vi "LeCroy Wave Series Acquire Waveform With Preview.vi"() -> ()   [LabVIEW 2018]
doc: "This example shows how to use advanced waveform readout parameters. The Preview Waveform Data graph shows signal decimated based on First Point, Sparsing and Number Of Points parameters. The Full Waveform Data graph shows full data as they were acquired by the instrument.\nObserve the time it takes to download the preview data and the full data."
uses:
  LeCroy Wave Series.lvlib
panel:
  in  "Number Of Points (0: all points)":i32
  in  "First Point (0: first point)":i32
  out "Full Download Time":u32
  out "Full Waveform Data":waveform(dbl)(graph)
  in  "Sparsing (1000)":i32=1000
  out "Preview Download Time":u32
  in  "Maximum Sample Points (1M)":i32(ring)=1000000 items=["50"=50, "100"=100, "250"=250, "500"=500, "1000"=1000, "2500"=2500, "5K"=5000, "10K"=10000, "25K"=25000, "50K"=50000, "100K"=100000, "250K"=250000, "500K"=500000, "1M"=1000000]
  in  "Vertical Coupling (0: A1M)":u16(ring) items=["A1M", "D1M", "D50", "Ground"]
  in  "Probe Attenuation (-1)":dbl=-1.0
  in  "Vertical Range (1.0 V)":dbl=10.0
  in  "Timebase (0.0005 s)":dbl=0.0005
  out "Preview Waveform Data":waveform(dbl)(graph)
  in  "Source (0: Channel 1)":u16(ring) items=["Channel 1", "Channel 2", "Channel 3", "Channel 4"]
  in  "VISA resource name":refnum<visa-resource-name>
  # "(c) 2005 - 2012 NATIONAL INSTRUMENTS.  ALL RIGHTS RESERVED."
  # "Note:\nThis VI will time out without acquiring any data if the input signal on channel 1 does not cross 0 V trigger level with positive slope.\nFor more details on triggering pleas see the Edge Triggered Acquisition Example VI."
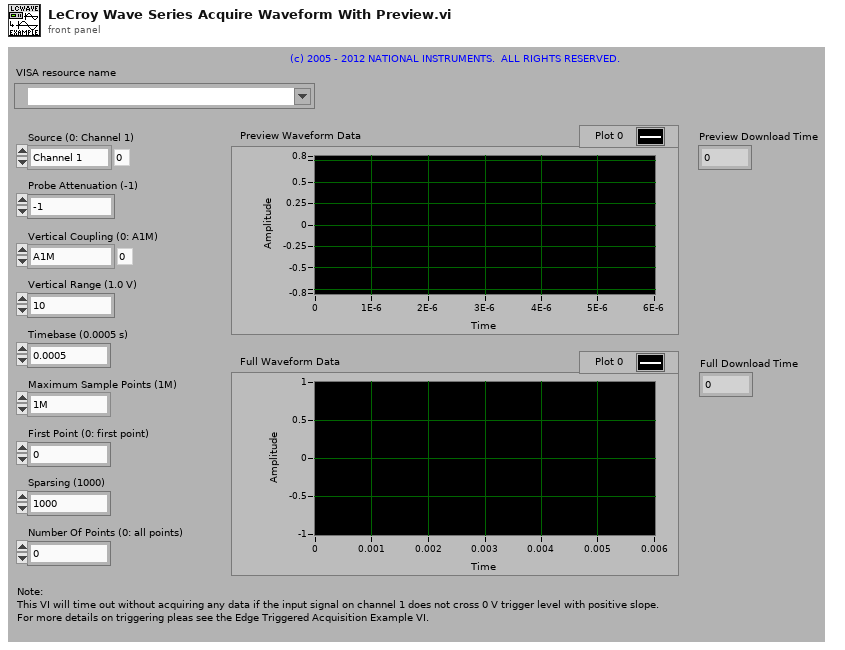
[diagram p1: front panel]
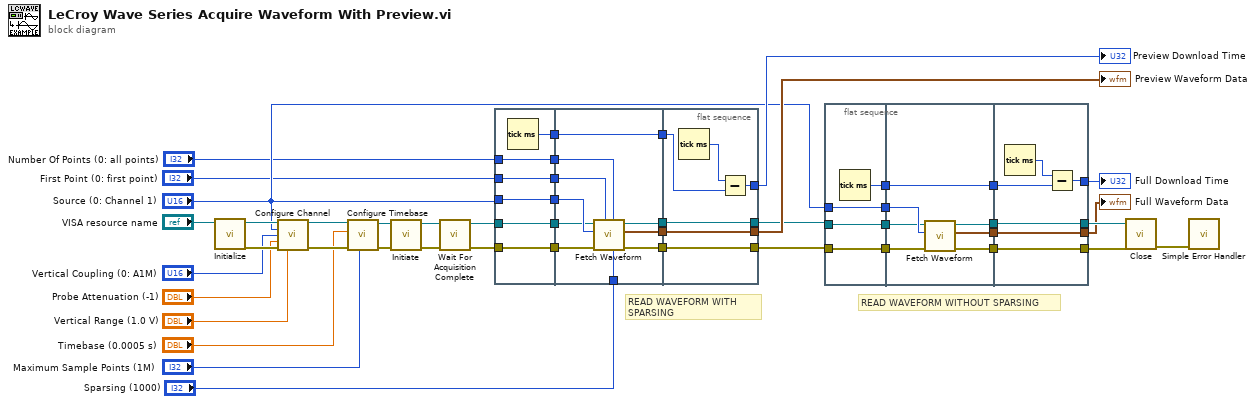
[diagram p0: block diagram]
diagram:
  # "READ WAVEFORM WITHOUT SPARSING"
  # "READ WAVEFORM WITH SPARSING"
  n1 = call "Initialize.vi"("VISA resource name"="VISA resource name") -> ("error out"=w41:errorcluster, "VISA resource name out"=w42:refnum<visa-resource-name>)  [unwired: 9 in]
  n2 = call "Configure Channel.vi"("VISA resource name"=w42, "Channel (0: Channel 1)"="Source (0: Channel 1)", "Vertical Coupling (0: A1M)"="Vertical Coupling (0: A1M)", "Probe Attenuation (-1.0)"="Probe Attenuation (-1)", "error in (no error)"=w41, "Vertical Range (10.0 V)"="Vertical Range (1.0 V)") -> ("VISA resource name out"=w45:refnum<visa-resource-name>, "error out"=w46:errorcluster)  [unwired: 8 in]
  n3 = call "Configure Timebase.vi"("Maximum Sample Points (500)"="Maximum Sample Points (1M)", "error in (no error)"=w46, "Timebase (0.0005 s)"="Timebase (0.0005 s)", "VISA resource name"=w45) -> ("error out"=w6:errorcluster, "VISA resource name out"=w5:refnum<visa-resource-name>)  [unwired: 6 in]
  n4 = call "Initiate.vi"("error in (no error)"=w6, "VISA resource name"=w5) -> ("error out"=w4:errorcluster, "VISA resource name out"=w3:refnum<visa-resource-name>)  [unwired: 8 in]
  n5 = call "Wait For Acquisition Complete.vi"("error in (no error)"=w4, "VISA resource name"=w3) -> ("error out"=w1:errorcluster, "VISA resource name out"=w2:refnum<visa-resource-name>)  [unwired: 7 in, 1 out]
  n6 = flat-sequence {
    tunnel: "Source (0: Channel 1)" -> [w52]
    tunnel: [w52] -> w18
    tunnel: w2 -> [w51]
    tunnel: [w51] -> w17
    tunnel: w1 -> [w50]
    tunnel: [w50] -> w16
    tunnel: "First Point (0: first point)" -> [w49]
    tunnel: [w49] -> w15
    tunnel: [w53] -> w14
    tunnel: [w48] -> w8
    tunnel: "Number Of Points (0: all points)" -> [w48]
    tunnel: [w63] -> w13
    tunnel: w18 -> [w62]
    tunnel: w17 -> [w61]
    tunnel: w16 -> [w60]
    tunnel: [w59] -> w12
    tunnel: [w58] -> w11
    tunnel: w15 -> [w57]
    tunnel: w14 -> [w56]
    tunnel: [w56] -> w10
    tunnel: "Sparsing (1000)" -> [w55]
    tunnel: w8 -> [w54]
    tunnel: [w66] -> w40
    tunnel: w13 -> [w66]
    tunnel: [w68] -> w35
    tunnel: [w65] -> w34
    tunnel: w12 -> [w65]
    tunnel: [w64] -> w33
    tunnel: w11 -> [w64]
    tunnel: w10 -> [w69]
    frame #0 {
      n7 = Tick Count (ms)() -> (millisecond timer value=w53:u32)
    }
    frame #1 {
      n8 = call "Fetch Waveform.vi"("Sparsing (0: Every point)"=w55, "Number of points (0: All points)"=w54, "First point (0: First point)"=w57, "error in (no error)"=w60, "Source (0: Channel 1)"=w62, "VISA resource name"=w61) -> ("error out"=w58:errorcluster, "Waveform Graph"=w63:waveform(dbl), "VISA resource name out"=w59:refnum<visa-resource-name>)  [unwired: 3 in]
    }
    frame #2 {
      n9 = Tick Count (ms)() -> (millisecond timer value=w67:u32)
      n10 = Subtract(x=w67, y=w69) -> (x-y=w68:u32)
    }
  }
  n11 = flat-sequence {
    tunnel: "Source (0: Channel 1)" -> [w72]
    tunnel: [w72] -> w26
    tunnel: w34 -> [w71]
    tunnel: [w71] -> w25
    tunnel: w33 -> [w70]
    tunnel: [w70] -> w24
    tunnel: [w73] -> w23
    tunnel: [w80] -> w22
    tunnel: w26 -> [w79]
    tunnel: w25 -> [w78]
    tunnel: w24 -> [w77]
    tunnel: [w76] -> w21
    tunnel: [w75] -> w20
    tunnel: w23 -> [w74]
    tunnel: [w74] -> w19
    tunnel: [w83] -> w29
    tunnel: w22 -> [w83]
    tunnel: [w85] -> w28
    tunnel: [w82] -> w32
    tunnel: w21 -> [w82]
    tunnel: [w81] -> w31
    tunnel: w20 -> [w81]
    tunnel: w19 -> [w86]
    frame #0 {
      n12 = Tick Count (ms)() -> (millisecond timer value=w73:u32)
    }
    frame #1 {
      n13 = call "Fetch Waveform.vi"("error in (no error)"=w77, "Source (0: Channel 1)"=w79, "VISA resource name"=w78) -> ("error out"=w75:errorcluster, "Waveform Graph"=w80:waveform(dbl), "VISA resource name out"=w76:refnum<visa-resource-name>)  [unwired: 6 in]
    }
    frame #2 {
      n14 = Tick Count (ms)() -> (millisecond timer value=w84:u32)
      n15 = Subtract(x=w84, y=w86) -> (x-y=w85:u32)
    }
  }
  n16 = call "Close.vi"("error in (no error)"=w31, "VISA resource name"=w32) -> ("error out"=w47:errorcluster)  [unwired: 9 in]
  n17 = call <vilib>:"Simple Error Handler.vi"("error in (no error)"=w47) -> ()  [unwired: 4 in, 5 out]
  "Preview Waveform Data" <- w40
  "Preview Download Time" <- w35
  "Full Waveform Data" <- w29
  "Full Download Time" <- w28
